vi "FIR Filter For Rational Resample.vi"(8 "anti-aliasing?":bool, 9 "FIR filter specifications":T1={"alias rejection (dB)"=120.0, "normalized bandwidth"=0.4536} {"normalized bandwidth" format="%.4f"; "alias rejection (dB)" format="%.2f"}, 10 "start index":i32, 11 "resample factor":cluster{"interpolation":i32, "decimation":i32}) -> (0 "error":i32, 1 "start index out":i32, 2 "decimation":i32, 3 "interpolation out":i32, 4 "filter coefficients":dbl[](array[numeric]) format="%.2f")   [LabVIEW 2020, in "NI_AALPro.lvlib"]
uses:
  <vilib>/Analysis/NI_AALPro.lvlib
  <vilib>/gmath/NI_Gmath.lvlib
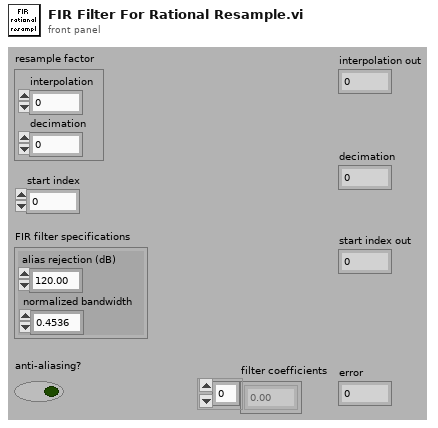
[diagram p1: front panel]
types:
  T1 = cluster{"alias rejection (dB)":dbl, "normalized bandwidth":dbl}
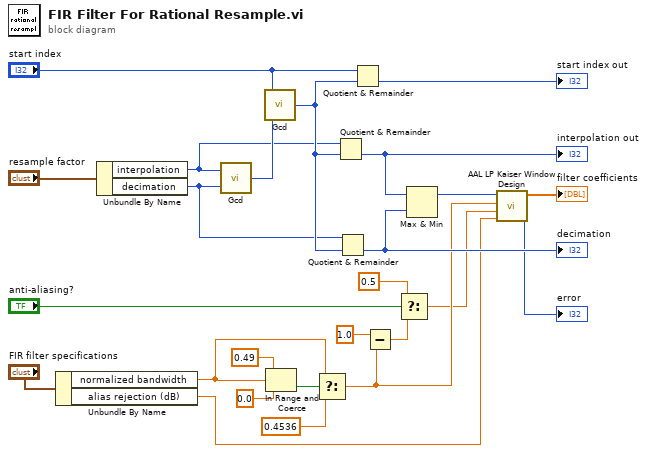
[diagram p0: block diagram]
diagram:
  n1 = Unbundle By Name("FIR filter specifications") -> ("normalized bandwidth"=w8:dbl, "alias rejection (dB)"=w3:dbl)
  n2 = Unbundle By Name("resample factor") -> ("interpolation"=w12:i32, "decimation"=w11:i32)
  n3 = call <vilib>:"Gcd.vi"("y"=w11, "x"=w12) -> ("gcd(x,y)"=w14:i32)
  n4 = call <vilib>:"Gcd.vi"("y"=w14, "x"="start index") -> ("gcd(x,y)"=w13:i32)
  n5 = In Range and Coerce(upper limit=0.49, x=w8, lower limit=0.0) -> (In Range?=w10:bool)  [unwired: 1 out]
  n6 = Select(t=w8, s=w10, f=0.4536 ("upper limit")) -> (s? t:f=w2:dbl)
  n7 = Quotient & Remainder(x=w12, y=w13) -> (floor(x/y)=w25:i32)  [unwired: 1 out]
  "interpolation out" <- w25
  n8 = Quotient & Remainder(x=w11, y=w13) -> (floor(x/y)=w24:i32)  [unwired: 1 out]
  "decimation" <- w24
  n9 = Quotient & Remainder(x="start index", y=w13) -> (floor(x/y)=→"start index out":i32)  [unwired: 1 out]
  n10 = Subtract(x=1.0, y=w2) -> (x-y=w4:dbl)
  n11 = Select(t=0.5 ("upper limit"), s="anti-aliasing?", f=w4) -> (s? t:f=w1:dbl)
  n12 = Max & Min(x=w25, y=w24) -> (max(x,y)=w15:i32)  [unwired: 1 out]
  n13 = call <vilib>:"AAL LP Kaiser Window Design.vi"("A stop [dB]"=w3, "stopband"=w1, "passband"=w2, "fs"=w15) -> ("error"=→"error":i32, "filter coefficients"=→"filter coefficients":dbl[])  [unwired: 5 in, 1 out]
